vi "setShutterMode.vi"(11 "mode":T1) -> ()   [LabVIEW 2016]
uses:
  <userlib>/atmcd64d.llb/Shutter_mode typedef.ctl
  <userlib>/atmcd64d.llb/Shutter_type typedef.ctl
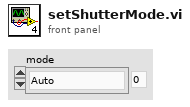
[diagram p1: front panel]
types:
  T1 = typedef "Shutter_mode typedef.ctl" = enum16{"Auto", "Close", "Open", "N/A (3)", "Open FVB Series", "Open Any Series"}
  T2 = typedef "Shutter_type typedef.ctl" = enum16{"TTL Low", "TTL High"}
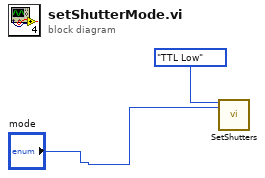
[diagram p0: block diagram]
diagram:
  n1 = call <userlib>:"SetShutters.vi"("type"=Shutter_type_typedef."TTL Low", "mode"="mode") -> ()  [unwired: 16 in, 2 out]
